vi "StrArray to CatStr.vi"(1 "String Array":string[](array[string])) -> (0 "spreadsheet string":string)   [LabVIEW 2019]
panel:
  out "number of replacements":i32
  out "result string":string
  out "spreadsheet string 2":string
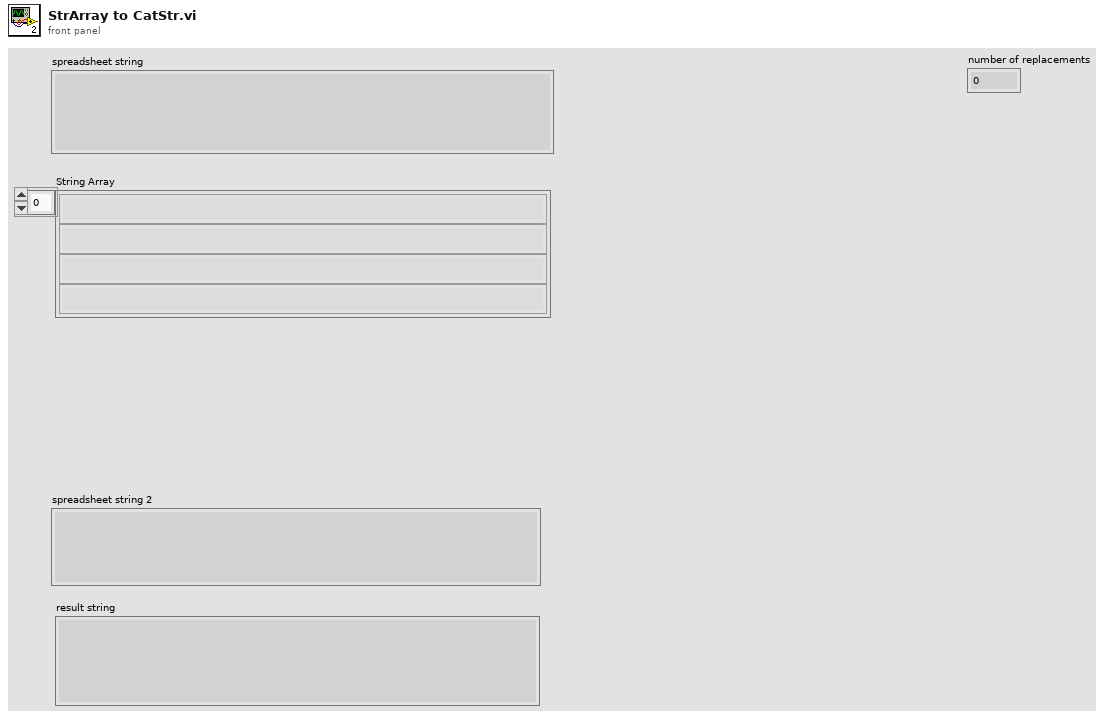
[diagram p1: front panel]
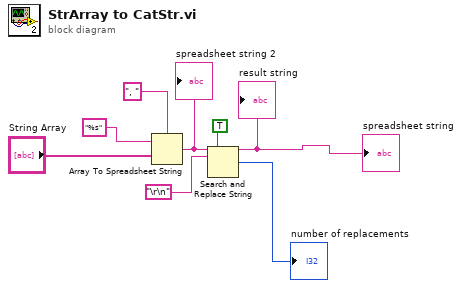
[diagram p0: block diagram]
diagram:
  n1 = Array To Spreadsheet String(delimiter (Tab)=", ", array="String Array", 3:"%s" ("format string")) -> (spreadsheet string=w5:string)
  "spreadsheet string 2" <- w5
  n2 = Search and Replace String(replace all?=TRUE ("replace all? (F)"), input string=w5, search string="\r\n") -> (result string=→"spreadsheet string" →"result string":string, number of replacements=→"number of replacements":i32)  [unwired: 5 in, 2 out]
